vi "zapishistorii.vi"() -> (3 "appended path":path)   [LabVIEW 2012]
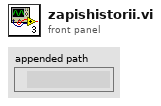
[diagram p1: front panel]
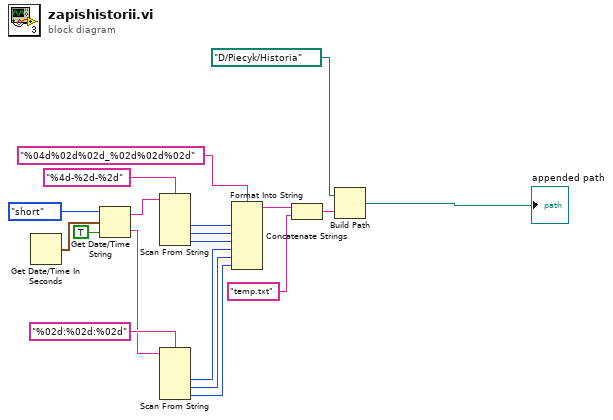
[diagram p0: block diagram]
diagram:
  n1 = Get Date/Time In Seconds() -> (seconds since 1Jan1904=w2:timestamp)
  n2 = Get Date/Time String(date format (0)=enum16{"short", "long", "abbreviated"}."short", seconds (now)=w2, want seconds? (F)=TRUE) -> (date string=w4:string, time string=w6:string)
  n3 = Scan From String(format string="%4d-%2d-%2d", input string=w4) -> (output 1=w8:i32, output 2=w9:i32, output 3=w10:i32)  [unwired: 5 in, 3 out]
  n4 = Scan From String(format string="%02d:%02d:%02d", input string=w6) -> (output 1=w12:i32, output 2=w13:i32, output 3=w14:i32)  [unwired: 5 in, 3 out]
  n5 = Format Into String(format string="%04d%02d%02d_%02d%02d%02d", w8, w9, w10, w12, w13, w14) -> (resulting string=w15:string)  [unwired: 2 in, 1 out]
  n6 = Concatenate Strings(w15, "temp.txt" ("string")) -> (w18:string)
  n7 = Build Path(base path=path "D:/Piecyk/Historia", name or relative path=w18) -> (appended path=→"appended path":path)
